vi "MIU_LeakTest.vi"() -> ()   [LabVIEW 2010]
uses:
  <vilib>/Utility/error.llb/DialogType.ctl
  <vilib>/Instr/_visa.llb/VISA Configure Serial Port (Instr).vi
  <vilib>/Analysis/NI_AALPro.lvlib
panel:
  in  "8 Port / 16 Port":i32=8
  in  "ValveSwitch Delay":u32=90
  out "PRESSURE":string="0"
  out "PRESSURE":dbl(graph)=80.268
  in  "Control Port":refnum<visa-resource-name>="COM4"
  in  "Control baud rate":u32=9600
  out "Time":string="0"
  out "Date":string="0"
  in  "Serial Read Port":refnum<visa-resource-name>="COM5"
  in  "data bits":u16=8 min=5 max=8 step=1
  in  "parity":u16(ring) items=["None", "Odd", "Even", "Mark", "Space"]
  in  "stop bits":u16(ring)=10 items=["1.0"=10, "1.5"=15, "2.0"=20]
  in  "flow control":u16(ring) items=["None"=0, "XON/XOFF"=1, "RTS/CTS"=2, "DTR/DSR"=4]
  in  "delay before read (ms)":u32=500
  in  "byte count":u32=500
  out "return count":u32
  in  "Instrument baud rate (9600)":u32=9600
  in  "stop":bool
  out "Pressure Leak Rate":cluster{i32[], "Best Linear Fit":dbl[]}[](graph)
  out "Leak Rate":dbl
  in  "Points to Average":i32=30
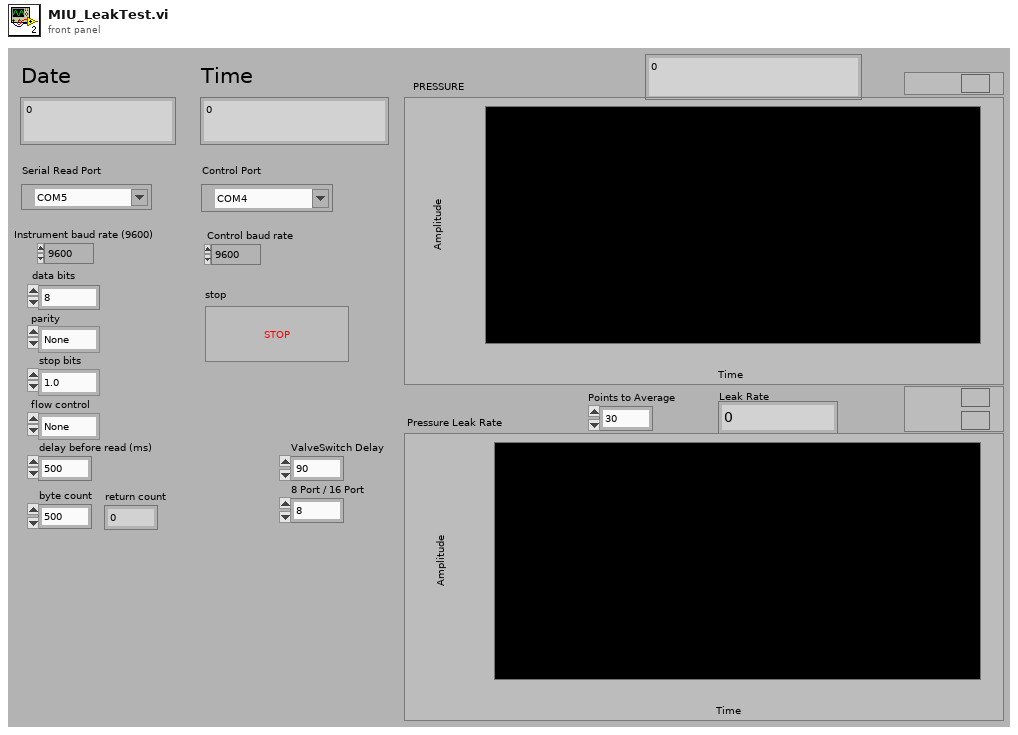
[diagram p1: front panel]
types:
  T1 = typedef "DialogType.ctl" = u16
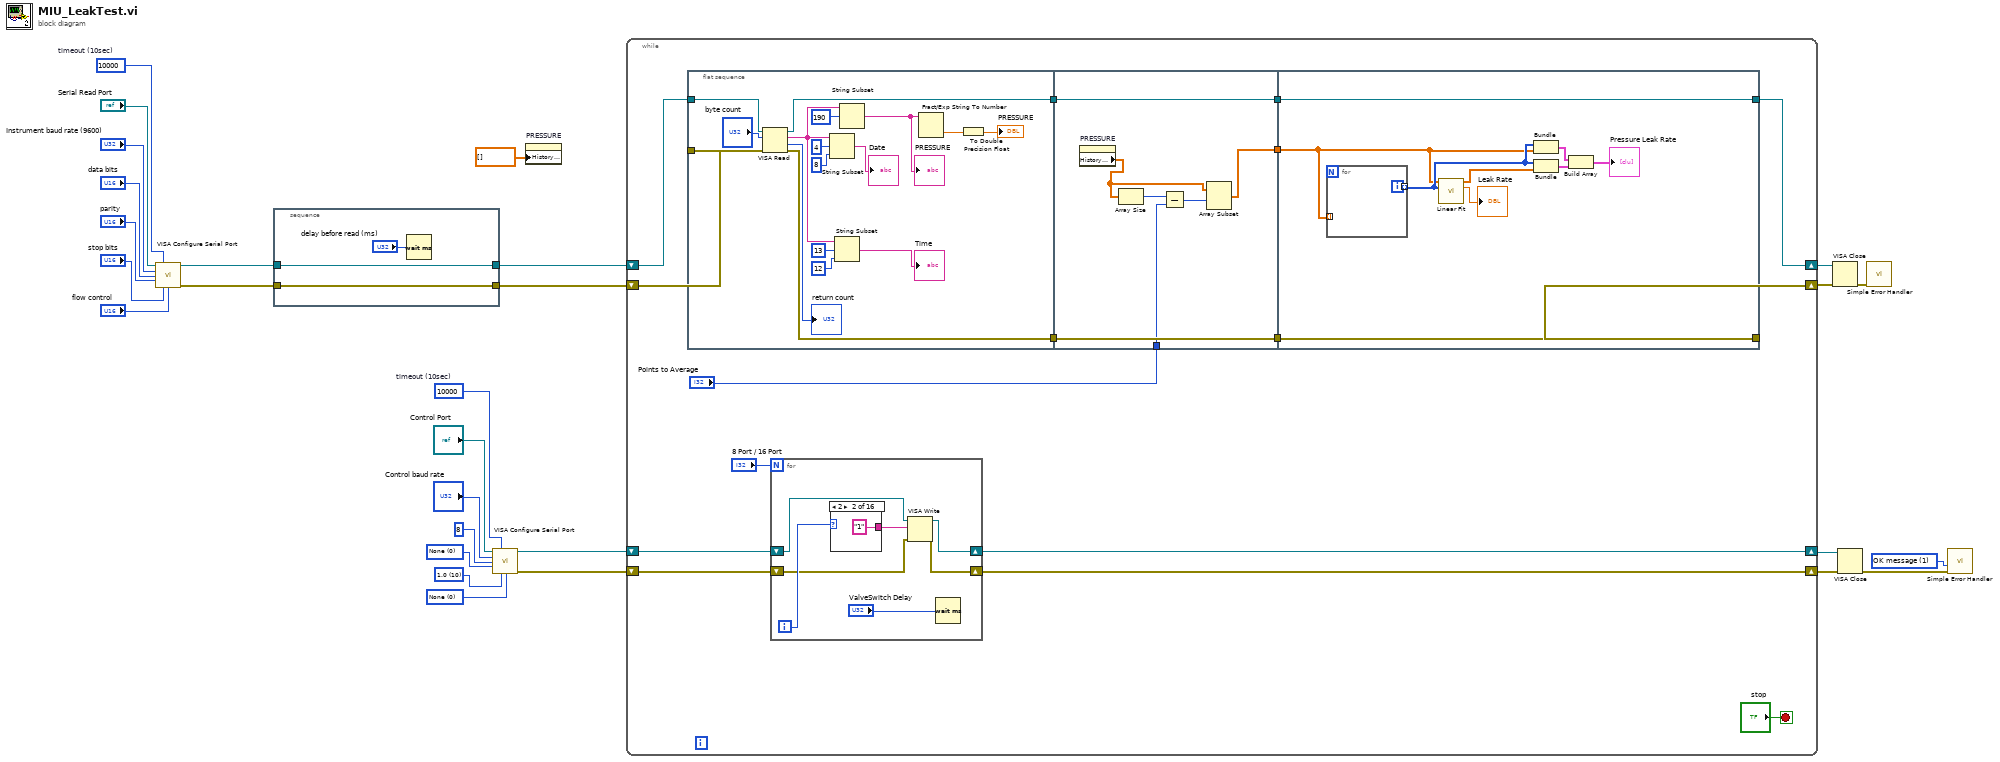
[diagram p0: block diagram]
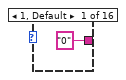
[diagram p2: hidden frame]
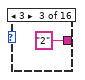
[diagram p3: hidden frame]
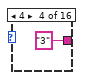
[diagram p4: hidden frame]
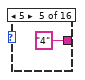
[diagram p5: hidden frame]
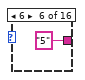
[diagram p6: hidden frame]
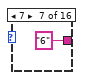
[diagram p7: hidden frame]
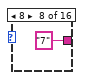
[diagram p8: hidden frame]
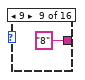
[diagram p9: hidden frame]
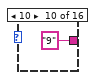
[diagram p10: hidden frame]
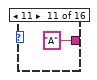
[diagram p11: hidden frame]
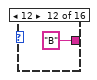
[diagram p12: hidden frame]
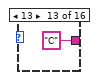
[diagram p13: hidden frame]
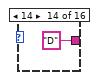
[diagram p14: hidden frame]
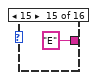
[diagram p15: hidden frame]
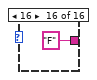
[diagram p16: hidden frame]
diagram:
  w7 = T1 1 items=["no dialog", "OK message", "continue or stop message", "OK message + warnings", "continue/stop + warnings"] ("type of dialog (OK msg:1)")
  w11 = u16 0 items=["None"=0, "XON/XOFF"=1, "RTS/CTS"=2, "DTR/DSR"=4] ("flow control")
  w12 = u16 10 items=["1.0"=10, "1.5"=15, "2.0"=20] ("stop bits")
  w14 = u16 0 items=["None", "Odd", "Even", "Mark", "Space"] ("parity")
  w13 = u32 10000  # timeout (10sec)
  w25 = u32 10000  # timeout (10sec)
  n1 = call-poly "VISA Configure Serial Port"("VISA resource name"="Serial Read Port", "timeout (10sec)"=w25, "baud rate (9600)"="Instrument baud rate (9600)", "data bits (8)"="data bits", "parity (0:none)"="parity", "stop bits (10: 1 bit)"="stop bits", "flow control (0:none)"="flow control") -> ("VISA resource name out"=w20:refnum<visa-resource-name>, "error out"=w21:errorcluster)  [unwired: 2 in, 5 out]
  n2 = stacked-sequence {
    tunnel: w21 -> [w31]
    tunnel: [w31] -> w1
    tunnel: w20 -> [w30]
    tunnel: [w30] -> w2
    frame #0 {
      n3 = Wait (ms)(milliseconds to wait="delay before read (ms)") -> ()  [unwired: 1 out]
    }
  }
  n4 = call-poly "VISA Configure Serial Port"("VISA resource name"="Control Port", "timeout (10sec)"=w13, "baud rate (9600)"="Control baud rate", "data bits (8)"=u16 8 ("data bits"), "parity (0:none)"=w14, "stop bits (10: 1 bit)"=w12, "flow control (0:none)"=w11) -> ("VISA resource name out"=w6:refnum<visa-resource-name>, "error out"=w5:errorcluster)  [unwired: 2 in, 5 out]
  n5 = property on="PRESSURE" class="WFChart (strict)"("History Data"=dbl[] []) -> ()  [unwired: 2 in, 2 out]
  n6 = while {
    shift-right: [w35] -> w4
    shift-left: w6 -> [w37]
    shift-right: [w34] -> w3
    shift-left: w5 -> [w36]
    shift-right: [w47] -> w19
    shift-left: w2 -> [w44]
    shift-right: [w46] -> w18
    shift-left: w1 -> [w45]
    stop <- "stop" stop-if-true
    n7 = flat-sequence {
      tunnel: w45 -> [w72]
      tunnel: w44 -> [w71]
      tunnel: [w81] -> w43
      tunnel: [w74] -> w42
      tunnel: w43 -> [w94]
      tunnel: w42 -> [w93]
      tunnel: "Points to Average" -> [w89]
      tunnel: [w94] -> w40
      tunnel: [w93] -> w39
      tunnel: [w88] -> w38
      tunnel: [w102] -> w46
      tunnel: [w103] -> w47
      tunnel: w40 -> [w103]
      tunnel: w39 -> [w102]
      tunnel: w38 -> [w95]
      frame #0 {
        n8 = VISA Read(VISA resource name=w71, byte count="byte count", error in (no error)=w72) -> (VISA resource name out=w81:refnum<visa-resource-name>, read buffer=w77:string, return count=→"return count":u32, error out=w74:errorcluster)
        n9 = String Subset(string=w77, offset (0)=4, length (rest)=8 ("length (rest)")) -> (substring=→"Date":string)
        n10 = String Subset(string=w77, offset (0)=13, length (rest)=12 ("length (rest)")) -> (substring=→"Time":string)
        n11 = String Subset(string=w77, offset (0)=190) -> (substring=w78:string)  [unwired: 1 in]
        "PRESSURE" <- w78
        n12 = Fract/Exp String To Number(string=w78) -> (number=w79:dbl)  [unwired: 3 in, 1 out]
        n13 = To Double Precision Float(number=w79) -> (double precision float=→"PRESSURE":dbl)
      }
      frame #1 {
        n14 = property on="PRESSURE" class="WFChart (strict)"() -> ("History Data"=w90:dbl[])  [unwired: 2 in, 2 out]
        n15 = Array Size(array=w90) -> (size(s)=w91:i32)
        n16 = Subtract(x=w91, y=w89) -> (x-y=w92:i32)
        n17 = Array Subset(array=w90, index=w92) -> (w88:dbl[])  [unwired: 1 in]
      }
      frame #2 {
        n18 = for {
          tunnel: [w104] -> w101 mode=indexing
          tunnel: w95 -> [_] mode=indexing
          i -> [w104]
        }
        n19 = call <vilib>:"Linear Fit.vi"("Y"=w95, "X"=w101) -> ("Best Linear Fit"=w100:dbl[], "slope"=→"Leak Rate":dbl)  [unwired: 9 in, 3 out]
        n20 = Bundle(w101, w95) -> (w99:cluster{i32[], dbl[]})  [unwired: 1 in]
        n21 = Bundle(w101, "Best Linear Fit"=w100) -> (w98:cluster{i32[], "Best Linear Fit":dbl[]})  [unwired: 1 in]
        n22 = Build Array(w99, w98) -> (→"Pressure Leak Rate":cluster{i32[], "Best Linear Fit":dbl[]}[])
      }
    }
    n23 = for {
      N: "8 Port / 16 Port" -> [_]
      shift-right: [w50] -> w35
      shift-left: w37 -> [w52]
      shift-right: [w49] -> w34
      shift-left: w36 -> [w51]
      i -> [w53]
      n24 = case shown="2" w53 {
        tunnel: ["0" "1" "2" "3" "4" "5" "6" "7" "8" "9" "A" "B" "C" "D" "E" "F"] -> w54
        frame 1, Default {
        }
        frame 2 {
        }
        frame 3 {
        }
        frame 4 {
        }
        frame 5 {
        }
        frame 6 {
        }
        frame 7 {
        }
        frame 8 {
        }
        frame 9 {
        }
        frame 10 {
        }
        frame 11 {
        }
        frame 12 {
        }
        frame 13 {
        }
        frame 14 {
        }
        frame 15 {
        }
        frame 16 {
        }
      }
      n25 = VISA Write(VISA resource name=w52, write buffer=w54, error in (no error)=w51) -> (VISA resource name out=w50:refnum<visa-resource-name>, error out=w49:errorcluster)  [unwired: 1 out]
      n26 = Wait (ms)(milliseconds to wait="ValveSwitch Delay") -> ()  [unwired: 1 out]
    }
  }
  n27 = VISA Close(VISA resource name=w19, error in (no error)=w18) -> (error out=w27:errorcluster)
  n28 = VISA Close(VISA resource name=w4, error in (no error)=w3) -> (error out=w9:errorcluster)
  n29 = call <vilib>:"Simple Error Handler.vi"("error in (no error)"=w27) -> ()  [unwired: 1 in, 8 out]
  n30 = call <vilib>:"Simple Error Handler.vi"("type of dialog (OK msg:1)"=w7, "error in (no error)"=w9) -> ()  [unwired: 8 out]
